vi "Magnet.vi"(8 "error in (no error)":errorcluster, 11 "Magnet in":refnum<class "Magnet.lvclass">) -> (0 "error out":errorcluster, 3 "Magnet out":refnum<class "Magnet.lvclass">)   [LabVIEW 2009, in "Magnet.lvclass"]
uses:
  Magnet.lvclass
  Global/GPIB Numbers.vi
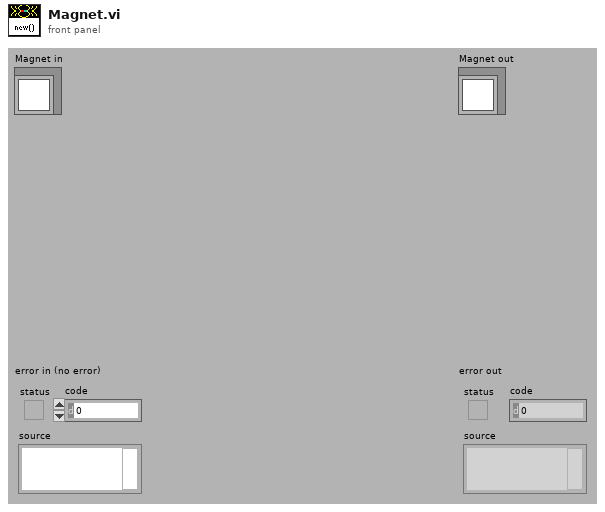
[diagram p1: front panel]
types:
  T1 = typedef "GPIB Type Def.ctl" = cluster{"Name":string, "bus":dbl, "GPIB":dbl, "GPIB as string":string, "byte":i32, "VISA Resource Name":refnum<visa-resource-name>}
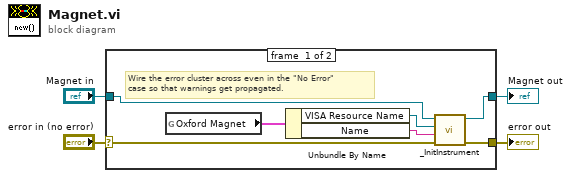
[diagram p0: block diagram]
diagram:
  n1 = case shown="No Error" "error in (no error)" {
    selector: "error in (no error)" -> [w9 w13]
    tunnel: [w8 w13] -> w3
    tunnel: [w10 w12] -> w1
    tunnel: "Magnet in" -> [w11 w12]
    frame #0 {
      # "Wire the error cluster across even in the \"No Error\"\ncase so that warnings get propagated."
      n2 = global read "GPIB Numbers.vi" "Oxford Magnet"() -> (w7:T1)
      n3 = Unbundle By Name(w7) -> ("VISA Resource Name"=w6:refnum<visa-resource-name>, "Name"=w5:string)
      n4 = call-dynamic "_InitInstrument.vi"("error in (no error)"=w9, "Name"=w5, "VISA Resource Name"=w6, "Instrument in"=w11) -> ("error out"=w8:errorcluster, "Instrument out"=w10:refnum<class "Magnet.lvclass">)  [unwired: 2 in, 4 out]
    }
    frame #1 {
    }
  }
  "error out" <- w3
  "Magnet out" <- w1
